vi "Voltage_overflow_checker.vi"(0 "Ch No":i32[](array[numeric]), 1 "Max":dbl=9.99, 2 "Voltages":dbl[][](array[numeric]), 3 "Ch Name":string[](array[string]), 4 "Min":dbl=-9.99) -> (5 "Over/Under string":string)   [LabVIEW 2017]
uses:
  Globals/Meas_global.vi
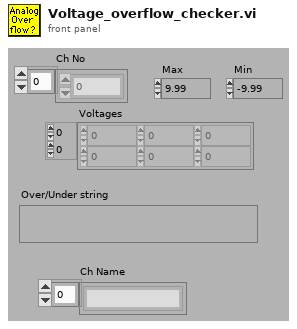
[diagram p1: front panel]
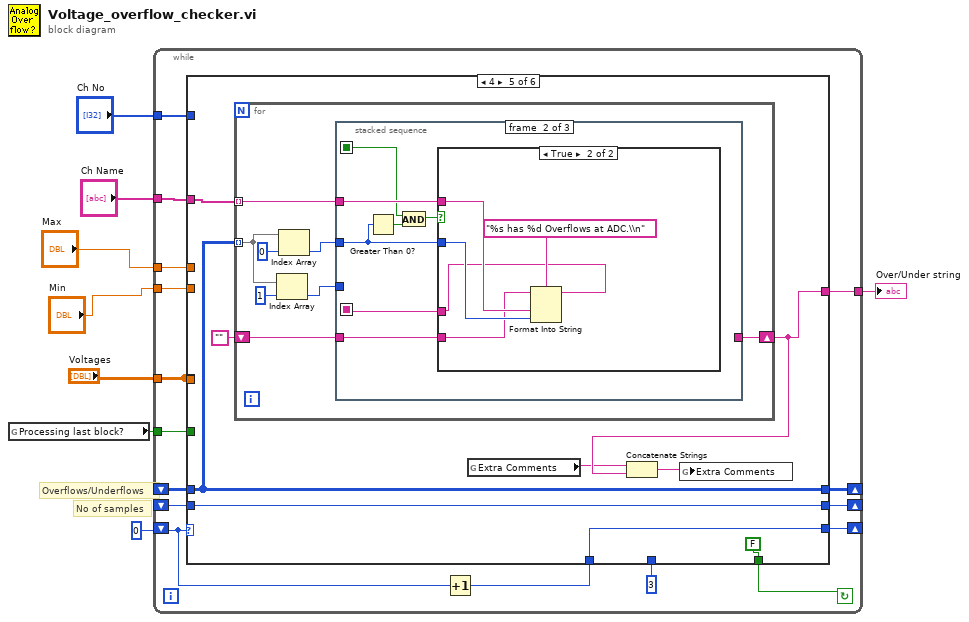
[diagram p0: block diagram]
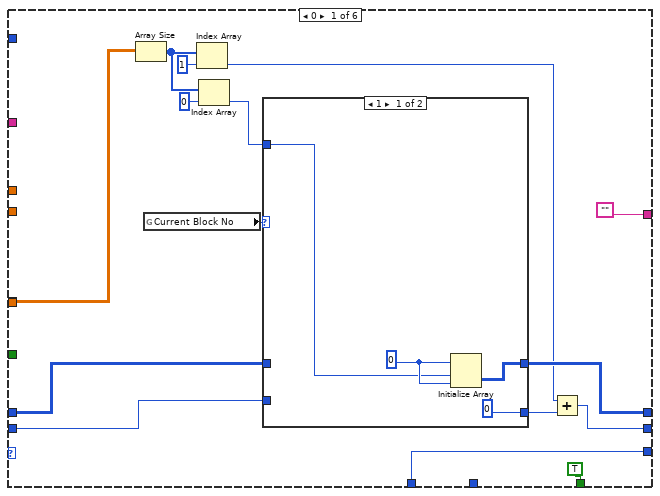
[diagram p2: hidden frame]
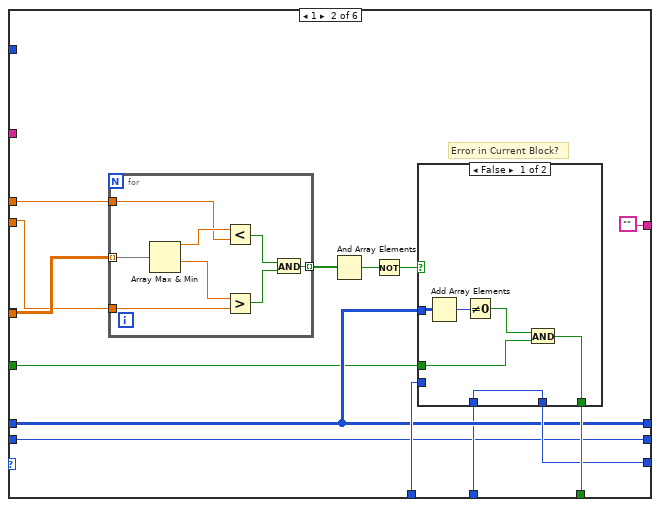
[diagram p4: hidden frame]
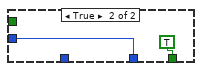
[diagram p5: hidden frame]
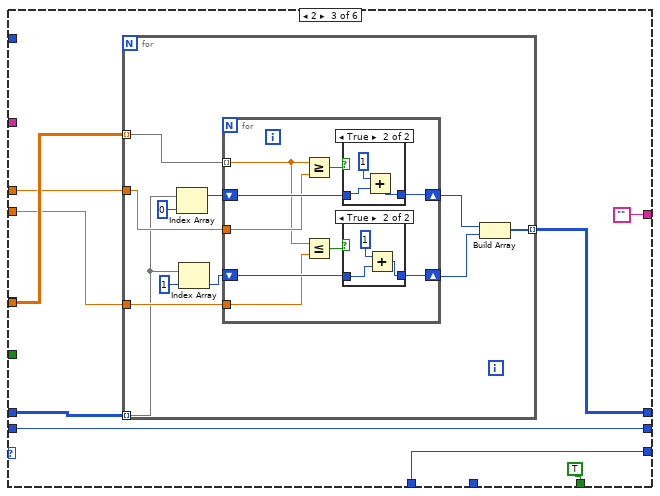
[diagram p6: hidden frame]
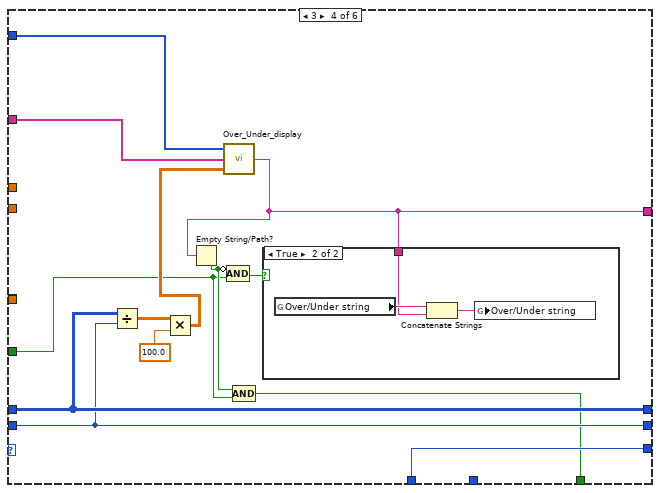
[diagram p9: hidden frame]
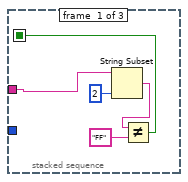
[diagram p11: hidden frame]
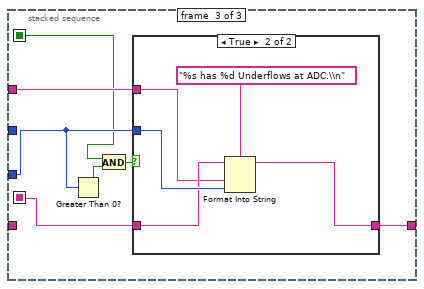
[diagram p13: hidden frame]
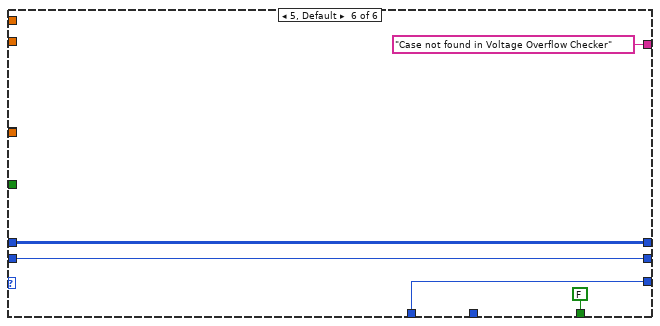
[diagram p15: hidden frame]
diagram:
  # "No of samples"
  # "Overflows/Underflows"
  n1 = global read "Meas_global.vi" "Processing last block?"() -> (w6:bool)
  n2 = while {
    tunnel: [w11] -> w5
    tunnel: w6 -> [w13]
    shift-left: _ -> [w17]
    shift-right: [w14] -> _
    shift-left: _ -> [w16]
    shift-right: [w15] -> _
    tunnel: "Voltages" -> [w18]
    shift-left: 0 -> [w21]
    shift-right: [w19] -> _
    tunnel: "Min" -> [w23]
    tunnel: "Max" -> [w24]
    tunnel: "Ch No" -> [w10]
    tunnel: "Ch Name" -> [w9]
    stop <- w22 continue-if-true
    n3 = Increment(x=w21) -> (x+1=w20:i32)
    n4 = case shown="4" w21 {
      tunnel: w24 -> [_ w58 w82 _ _ _]
      tunnel: w23 -> [_ w57 w83 _ _ _]
      tunnel: w18 -> [w31 w59 _ _ _ _]
      tunnel: [TRUE w54 TRUE w115 FALSE FALSE] -> w22
      tunnel: w20 -> [w34 w52 w80 w125 w137 w179]
      tunnel: [w34 w53 w80 w125 w137 w179] -> w19
      tunnel: w18 -> [_ _ w84 _ _ _]
      tunnel: w17 -> [w37 w48 w76 w123 w136 w180]
      tunnel: w16 -> [w35 w51 w77 w124 w133 w181]
      tunnel: [w38 w51 w81 w124 w133 w181] -> w15
      tunnel: [w28 w48 w76 w123 w136 w180] -> w14
      tunnel: w13 -> [_ w46 _ w116 _ _]
      tunnel: 3 -> [_ w50 _ _ _ _]
      tunnel: ["" "" "" w118 w131 "Case not found in Voltage Overflow Checker" ("Over/Under string")] -> w11
      tunnel: w10 -> [_ _ _ w114 _ _]
      tunnel: w9 -> [_ _ _ w113 w129 _]
      frame 0 {
        n5 = Array Size(array=w31) -> (size(s)=w26:i32[])
        n6 = global read "Meas_global.vi" "Current Block No"() -> (w39:i32)
        n7 = Index Array(array=w26, index=1 ("Index")) -> (element=w30:i32)
        n8 = Index Array(array=w26, index=0 ("Index")) -> (element=w25:i32)
        n9 = case shown="1" w39 {
          tunnel: [w43 w45] -> w38
          tunnel: w35 -> [_ w45]
          tunnel: w37 -> [_ w44]
          tunnel: [0 w44] -> w29
          tunnel: w25 -> [w40 _]
          frame 1 {
            w41 = 0
            n10 = Initialize Array(w41, w40, w41) -> (w43:i32[][])
          }
          frame 2, Default {
          }
        }
        n11 = Add(x=w30, y=w29) -> (x+y=w28:i32)
      }
      frame 1 {
        # "Error in Current Block?"
        n12 = for {
          tunnel: w59 -> [w75] mode=indexing
          tunnel: w58 -> [w73]
          tunnel: w57 -> [w71]
          tunnel: [w68] -> w56 mode=indexing
          n13 = Array Max & Min(array=w75) -> (max value=w74:dbl, min value=w72:dbl)  [unwired: 2 out]
          n14 = Less?(x=w74, y=w73) -> (x < y?=w69:bool)
          n15 = Greater?(x=w72, y=w71) -> (0:w70:bool)
          n16 = And(x=w69, y=w70) -> (x .and. y?=w68:bool)
        }
        n17 = And Array Elements(Boolean array=w56) -> (logical AND=w55:bool)
        n18 = Not(x=w55) -> (.not. x?=w47:bool)
        n19 = case shown="False" w47 {
          tunnel: [w61 TRUE] -> w54
          tunnel: [w60 w66] -> w53
          tunnel: w52 -> [_ w66]
          tunnel: w51 -> [w65 _]
          tunnel: w50 -> [w60 _]
          tunnel: w46 -> [w62 _]
          frame False {
            n20 = Add Array Elements(numeric array=w65) -> (sum=w64:i32)
            n21 = Not Equal To 0?(x=w64) -> (x != 0?=w63:bool)
            n22 = And(x=w63, y=w62) -> (x .and. y?=w61:bool)
          }
          frame True {
          }
        }
      }
      frame 2 {
        n23 = for {
          tunnel: w84 -> [w93] mode=indexing
          tunnel: w83 -> [w95]
          tunnel: w82 -> [w94]
          tunnel: [w91] -> w81 mode=indexing
          tunnel: w77 -> [w87] mode=indexing
          n24 = Index Array(array=w87, index=0 ("Index")) -> (element=w85:i32)
          n25 = Index Array(array=w87, index=1 ("Index")) -> (element=w86:i32)
          n26 = for {
            shift-right: [w99] -> w90
            shift-left: w86 -> [w100]
            shift-right: [w102] -> w92
            shift-left: w85 -> [w103]
            tunnel: w93 -> [w96] mode=indexing
            tunnel: w95 -> [w98]
            tunnel: w94 -> [w97]
            n27 = Greater Or Equal?(x=w96, y=w97) -> (x >= y?=w104:bool)
            n28 = Less Or Equal?(x=w96, y=w98) -> (x <= y?=w101:bool)
            n29 = case shown="True" w104 {
              tunnel: [w109 w111] -> w102
              tunnel: w103 -> [w109 w112]
              frame False {
              }
              frame True {
                n30 = Add(x=1, y=w112) -> (x+y=w111:i32)
              }
            }
            n31 = case shown="True" w101 {
              tunnel: w100 -> [w105 w107]
              tunnel: [w105 w106] -> w99
              frame False {
              }
              frame True {
                n32 = Add(x=1, y=w107) -> (x+y=w106:i32)
              }
            }
          }
          n33 = Build Array(w92, w90) -> (w91:i32[])
        }
      }
      frame 3 {
        n34 = Divide(x=w124, y=w123) -> (x/y=w122:dbl[][])
        n35 = Multiply(x=w122, y=100.0) -> (x*y=w120:dbl[][])
        n36 = call "Over_Under_display.vi"("Overflow array"=w120, "Ch Name"=w113, "Ch No"=w114) -> ("Over/Under string"=w118:string)
        n37 = Empty String/Path?(string/path=w118) -> (empty?=w117:bool)
        n38 = Compound Arithmetic op=AND(invert w117, w116) -> (w119:bool)
        n39 = Compound Arithmetic op=AND(w117, w116) -> (w115:bool)
        n40 = case shown="True" w119 {
          tunnel: w118 -> [_ w126]
          frame False {
          }
          frame True {
            n41 = global read "Meas_global.vi" "Over/Under string"() -> (w128:string)
            n42 = Concatenate Strings(w128, w126) -> (w127:string)
            n43 = global write "Meas_global.vi" "Over/Under string"(w127) -> ()
          }
        }
      }
      frame 4 {
        n44 = for {
          tunnel: w133 -> [w145] mode=indexing
          shift-right: [w139] -> w131
          shift-left: "" -> [w140]
          tunnel: w129 -> [w138] mode=indexing
          n45 = Index Array(array=w145, index=1) -> (element=w141:i32)
          n46 = Index Array(array=w145, index=0) -> (element=w142:i32)
          n47 = stacked-sequence {
            seq-local: [_ w155 _] -> [_ _ w170]
            seq-local: [w146 _ _] -> [_ w152 w164]
            tunnel: w141 -> [_ _ w168]
            tunnel: w142 -> [_ w154 _]
            tunnel: w138 -> [w147 w157 w167]
            tunnel: w140 -> [_ w156 _]
            tunnel: [_ _ w169] -> w139
            frame #0 {
              n48 = String Subset(string=w147, length (rest)=2 ("length (rest)")) -> (substring=w149:string)  [unwired: 1 out]
              n49 = Not Equal?(x=w149, y="FF") -> (x != y?=w146:bool)
            }
            frame #1 {
              n50 = Greater Than 0?(x=w154) -> (x > 0?=w153:bool)
              n51 = And(x=w152, y=w153) -> (x .and. y?=w151:bool)
              n52 = case shown="True" w151 {
                tunnel: w154 -> [_ w161]
                tunnel: w157 -> [_ w162]
                tunnel: w156 -> [w158 w160]
                tunnel: [w158 w159] -> w155
                frame False {
                }
                frame True {
                  n53 = Format Into String(format string="%s has %d Overflows at ADC.\\n" ("Format String"), initial string=w160, w162, w161) -> (resulting string=w159:string)  [unwired: 1 in, 1 out]
                }
              }
            }
            frame #2 {
              n54 = Greater Than 0?(x=w168) -> (x > 0?=w166:bool)
              n55 = And(x=w164, y=w166) -> (x .and. y?=w165:bool)
              n56 = case shown="True" w165 {
                tunnel: w168 -> [_ w176]
                tunnel: w167 -> [_ w172]
                tunnel: w170 -> [w171 w175]
                tunnel: [w171 w174] -> w169
                frame False {
                }
                frame True {
                  n57 = Format Into String(format string="%s has %d Underflows at ADC.\\n" ("Format String"), initial string=w175, w172, w176) -> (resulting string=w174:string)  [unwired: 1 in, 1 out]
                }
              }
            }
          }
        }
        n58 = global read "Meas_global.vi" "Extra Comments"() -> (w130:string)
        n59 = Concatenate Strings(w130, w131) -> (w134:string)
        n60 = global write "Meas_global.vi" "Extra Comments"(w134) -> ()
      }
      frame 5, Default {
      }
    }
  }
  "Over/Under string" <- w5
